vi "Read Start Index.vi"(8 "error in (no error)":errorcluster, 11 "Set Ratios Msg in":refnum<class "Set Ratios Msg.lvclass">) -> (0 "error out":errorcluster, 2 "Start Index":i32, 3 "Set Ratios Msg out":refnum<class "Set Ratios Msg.lvclass">)   [LabVIEW 2017, in "BNT_DAQmx.lvlib" / "Set Ratios Msg.lvclass"]
uses:
  Set Ratios Msg.lvclass
  Set Ratios Msg.lvclass/Set Ratios Msg.ctl
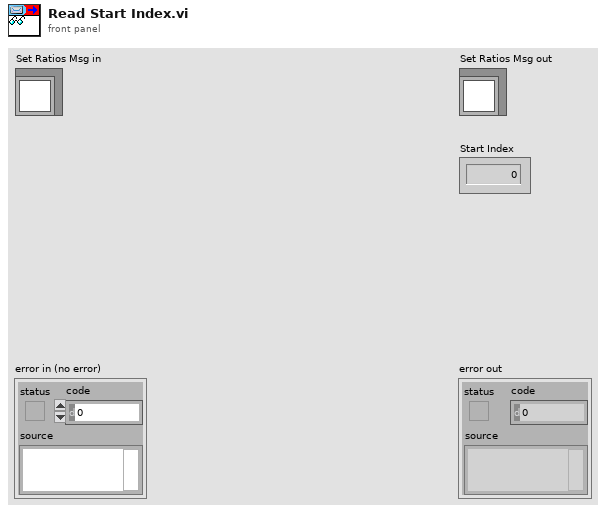
[diagram p1: front panel]
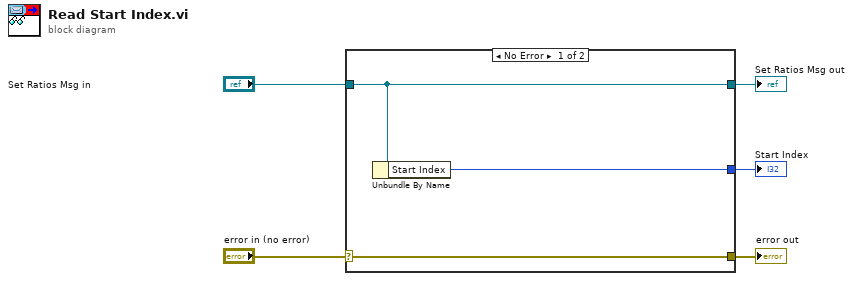
[diagram p0: block diagram]
diagram:
  n1 = case shown="No Error" "error in (no error)" {
    selector: "error in (no error)" -> [w8 w9]
    tunnel: [w8 w9] -> w4
    tunnel: [w7 w10] -> w2
    tunnel: "Set Ratios Msg in" -> [w7 w10]
    tunnel: [w6 _] -> w1
    frame No Error {
      n2 = Unbundle By Name(w7) -> ("Start Index"=w6:i32)
    }
    frame Error {
    }
  }
  "error out" <- w4
  "Set Ratios Msg out" <- w2
  "Start Index" <- w1
